vi "Digital Output.vi"(8 "error in":errorcluster, 11 "DAQmx OutPut Setting":T1) -> (0 "error out":errorcluster, 1 "Exit":bool)   [LabVIEW 2015]
uses:
  <vilib>/DAQmx/write.llb/DAQmx Write (Digital 2D Bool NChan 1Samp NLine).vi
  <vilib>/DAQmx/write.llb/DAQmx Write (Digital 1D Bool 1Chan 1Samp).vi
  <vilib>/DAQmx/create/channels.llb/DAQmx Create Channel (DO-Digital Output).vi
  Galobal variable_TI.vi
  <vilib>/DAQmx/miscellaneous.llb/DAQmx Fill In Error Info.vi
panel:
  out "error out 2":errorcluster
  out "array":tag[](array[tag])
  out "*(type *) &x":tag
  out "Digital Output":bool[](array[boolean])
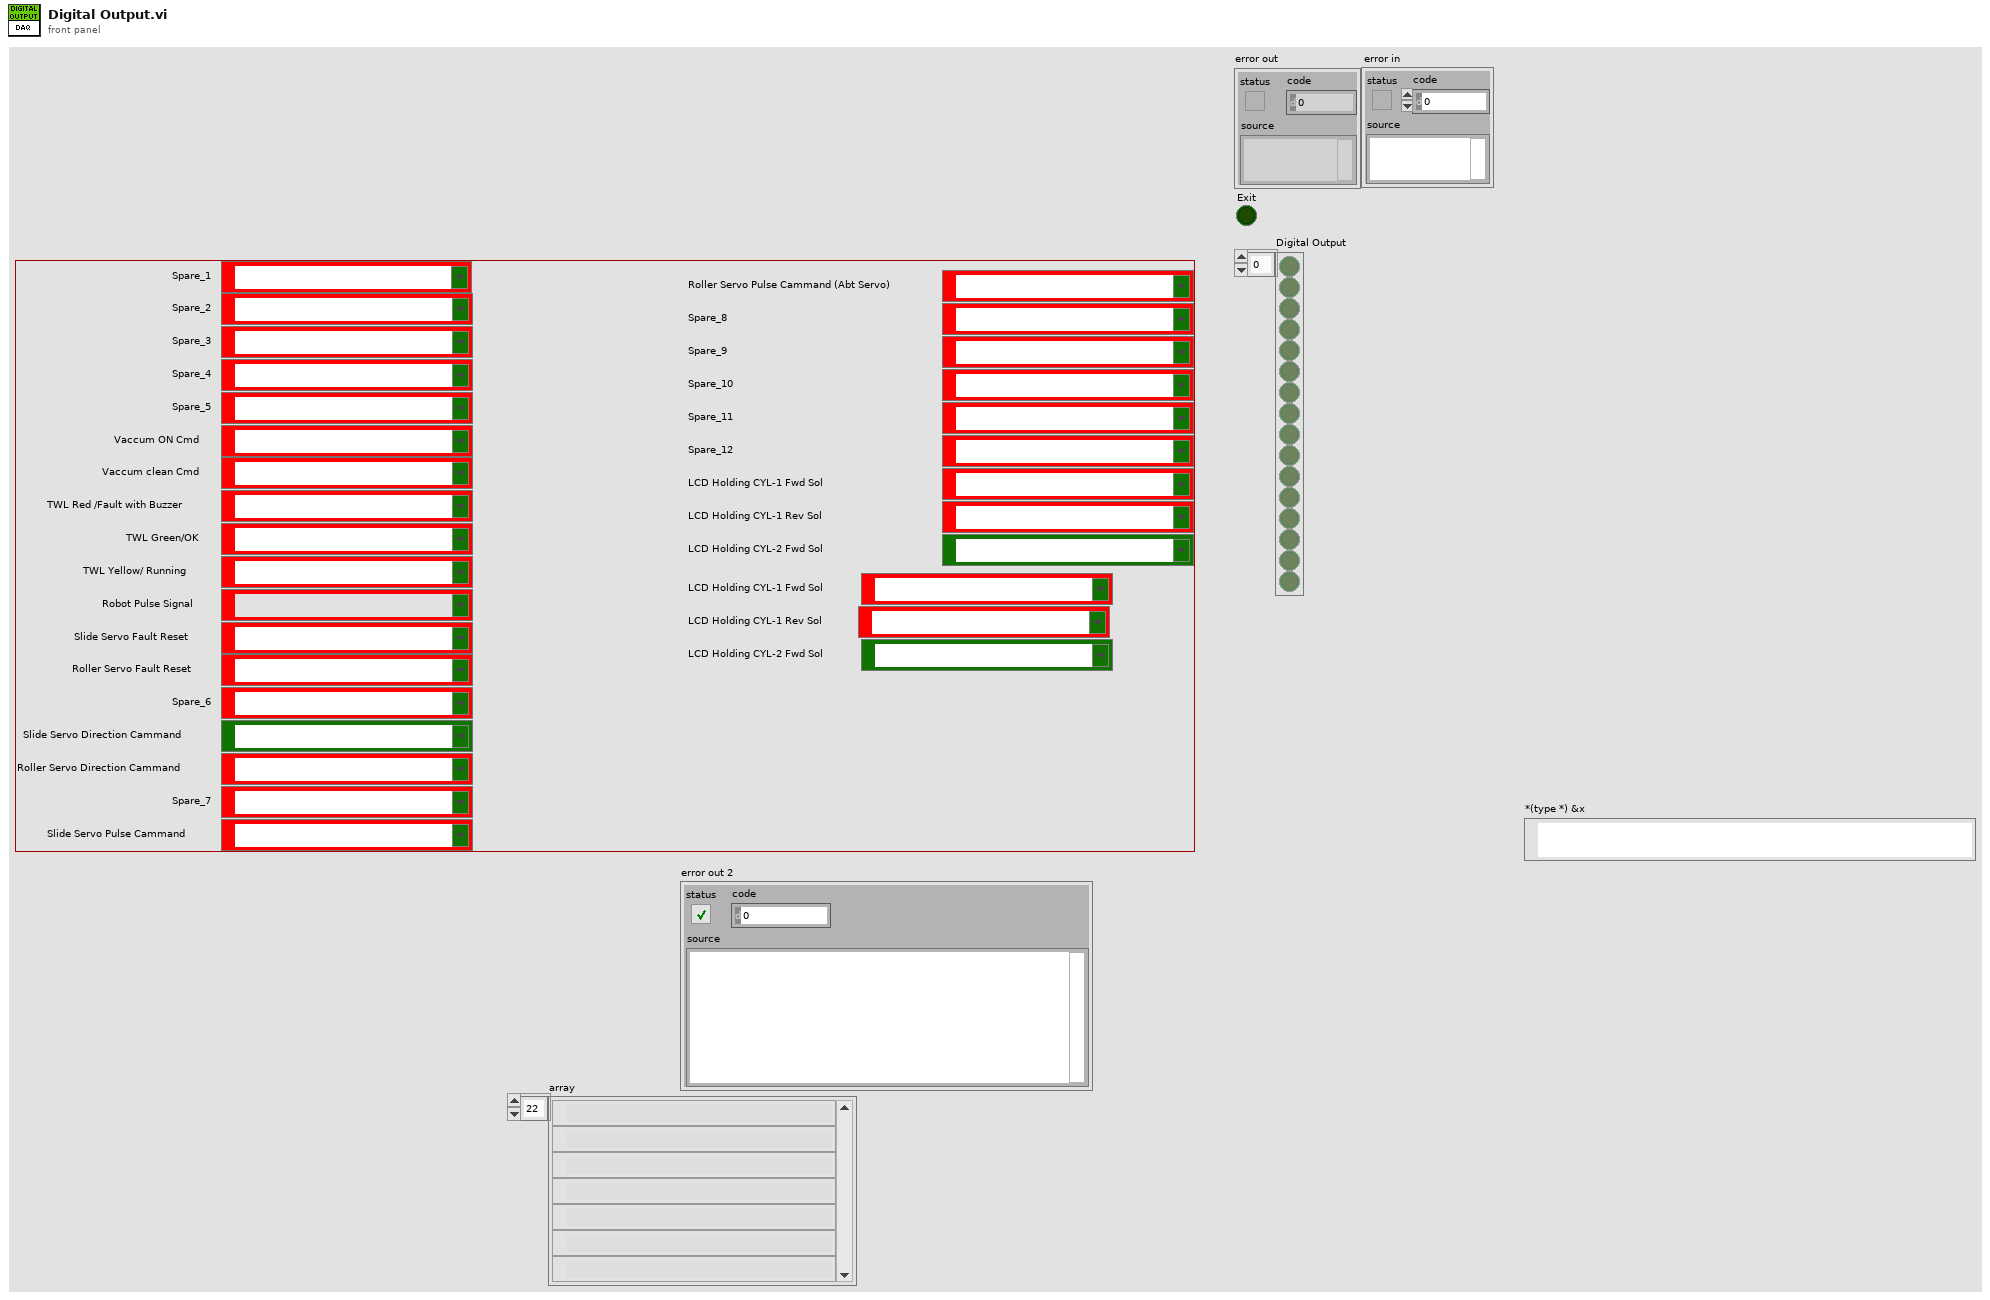
[diagram p1: front panel]
types:
  T1 = cluster{"DAQmx OutPut_00":tag, "DAQmx OutPut_01":tag, "DAQmx OutPut_02":tag, "DAQmx OutPut_03":tag, "DAQmx OutPut_04":tag, "DAQmx OutPut_05":tag, "DAQmx OutPut_06":tag, "DAQmx OutPut_07":tag, "DAQmx OutPut_08":tag, "DAQmx OutPut_09":tag, "DAQmx OutPut_10":tag, "DAQmx OutPut_11":tag, "DAQmx OutPut_12":tag, "DAQmx OutPut_13":tag, "DAQmx OutPut_14":tag, "DAQmx OutPut_15":tag, "DAQmx OutPut_16":tag, "DAQmx OutPut_17":tag, "DAQmx OutPut_18":tag, "DAQmx OutPut_19":tag, "DAQmx OutPut_20":tag, "DAQmx OutPut_21":tag, "DAQmx OutPut_22":tag, "DAQmx OutPut_23":tag, "DAQmx OutPut_12 2":tag, "DAQmx OutPut_13 2":tag, "DAQmx OutPut_14 2":tag, "DAQmx OutPut_12 3":tag, "DAQmx OutPut_13 3":tag, "DAQmx OutPut_14 3":tag}
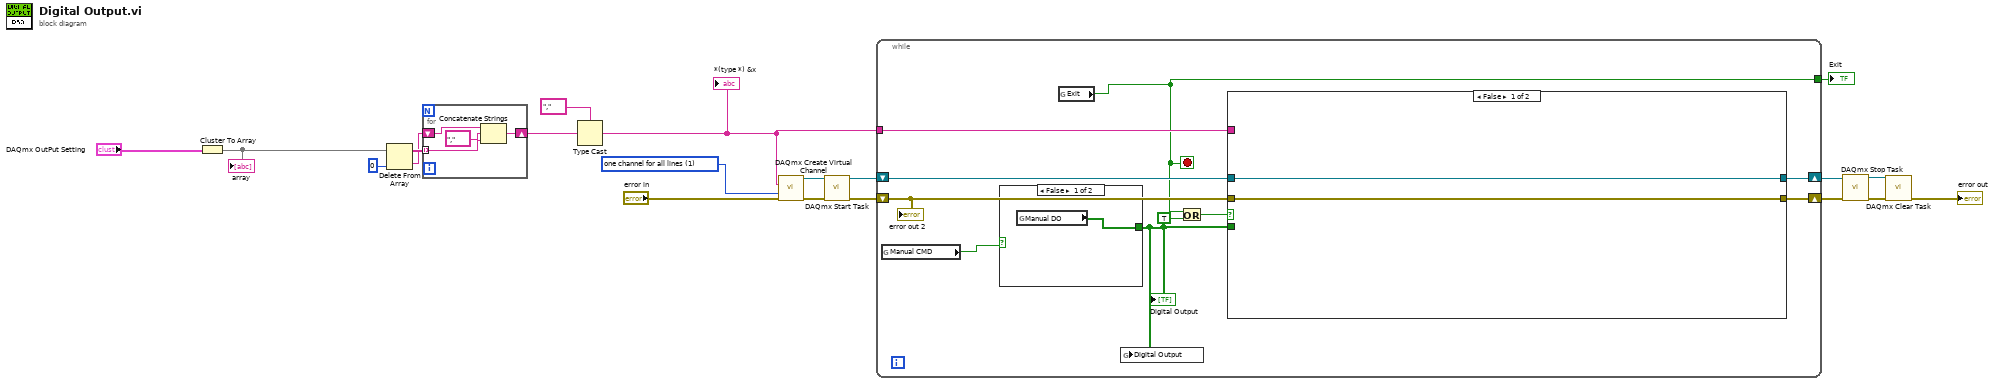
[diagram p0: block diagram]
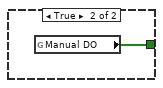
[diagram p2: hidden frame]
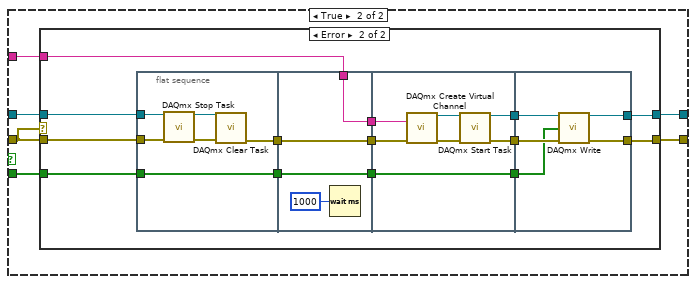
[diagram p3: hidden frame]
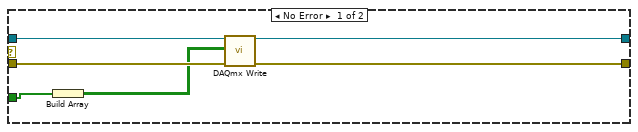
[diagram p4: hidden frame]
diagram:
  w4 = 1 items=["one channel for each line", "one channel for all lines"] ("line grouping")
  n1 = Cluster To Array(cluster="DAQmx OutPut Setting") -> (array=w2:tag[])
  "array" <- w2
  n2 = Delete From Array(array=w2, index=0) -> (deleted portion=w7:tag, array with subset deleted=w9:tag[])  [unwired: 1 in]
  n3 = for {
    tunnel: w9 -> [w23] mode=indexing
    shift-right: [w21] -> w5
    shift-left: w7 -> [w24]
    n4 = Concatenate Strings(w24, tag "," ("1."), w23) -> (w21:string)
  }
  n5 = Type Cast(type=tag "," ("1."), x=w5) -> (*(type *) &x=w3:tag)
  "*(type *) &x" <- w3
  n6 = call-poly <vilib>:"DAQmx Create Virtual Channel.vi"("lines"=w3, "line grouping"=w4, "error in"="error in") -> ("task out"=w20:refnum<k21>, "error out"=w19:errorcluster)  [unwired: 2 in, 9 out]
  n7 = call <vilib>:"DAQmx Start Task.vi"("task/channels in"=w20, "error in"=w19) -> ("task out"=w16:refnum<k21>, "error out"=w15:errorcluster)  [unwired: 12 out]
  n8 = while {
    shift-right: [w32] -> w13
    shift-left: w15 -> [w31]
    shift-right: [w33] -> w14
    shift-left: w16 -> [w34]
    tunnel: w3 -> [w30]
    tunnel: [w27] -> w10
    stop <- w27 stop-if-true
    n9 = global read "Galobal variable_TI.vi" "Manual CMD"() -> (w26:bool)
    n10 = case shown="False" w26 {
      tunnel: [w35 w36] -> w25
      frame False {
        n11 = global read "Galobal variable_TI.vi" "Manual DO"() -> (w35:bool[])
      }
      frame True {
        n12 = global read "Galobal variable_TI.vi" "Manual DO"() -> (w36:bool[])
      }
    }
    "Digital Output" <- w25
    n13 = global read "Galobal variable_TI.vi" "Exit"() -> (w27:bool)
    n14 = global write "Galobal variable_TI.vi" "Digital Output"(w25) -> ()
    n15 = Or(x=w27, y=TRUE) -> (x .or. y?=w29:bool)
    n16 = case shown="False" w29 {
      tunnel: w34 -> [w38 w44]
      tunnel: [w38 w43] -> w33
      tunnel: [w37 w42] -> w32
      tunnel: w31 -> [w37 w41]
      tunnel: w30 -> [_ w40]
      tunnel: w25 -> [_ w39]
      frame False {
      }
      frame True {
        n17 = case shown="Error" w41 {
          tunnel: w44 -> [w50 w64]
          tunnel: w41 -> [w49 w63]
          tunnel: [w48 w61] -> w43
          tunnel: [w47 w62] -> w42
          tunnel: w40 -> [_ w57]
          tunnel: w39 -> [w46 w54]
          frame No Error {
            n18 = Build Array(w46) -> (w45:bool[][])
            n19 = call-poly <vilib>:"DAQmx Write.vi"("task/channels in"=w50, "data"=w45, "error in"=w49) -> ("task out"=w48:refnum<k21>, "error out"=w47:errorcluster)  [unwired: 1 in, 10 out]
          }
          frame Error {
            n20 = flat-sequence {
              tunnel: w64 -> [w68]
              tunnel: w63 -> [w67]
              tunnel: [w66] -> w59
              tunnel: w54 -> [w65]
              tunnel: [w65] -> w53
              tunnel: [w73] -> w60
              tunnel: w59 -> [w73]
              tunnel: [w72] -> w58
              tunnel: w57 -> [w72]
              tunnel: w53 -> [w71]
              tunnel: [w71] -> w52
              tunnel: w60 -> [w77]
              tunnel: w58 -> [w76]
              tunnel: [w79] -> w56
              tunnel: [w78] -> w55
              tunnel: w52 -> [w75]
              tunnel: [w75] -> w51
              tunnel: [w84] -> w61
              tunnel: [w85] -> w62
              tunnel: w56 -> [w86]
              tunnel: w55 -> [w83]
              tunnel: w51 -> [w82]
              frame #0 {
                n21 = call <vilib>:"DAQmx Stop Task.vi"("task/channels in"=w68, "error in"=w67) -> ("task out"=w69:refnum<k21>, "error out"=w70:errorcluster)  [unwired: 12 out]
                n22 = call <vilib>:"DAQmx Clear Task.vi"("task in"=w69, "error in"=w70) -> ("error out"=w66:errorcluster)  [unwired: 13 out]
              }
              frame #1 {
                n23 = Wait (ms)(milliseconds to wait=u32 1000) -> ()  [unwired: 1 out]
              }
              frame #2 {
                n24 = call-poly <vilib>:"DAQmx Create Virtual Channel.vi"("lines"=w76, "error in"=w77) -> ("task out"=w81:refnum<k21>, "error out"=w80:errorcluster)  [unwired: 3 in, 9 out]
                n25 = call <vilib>:"DAQmx Start Task.vi"("task/channels in"=w81, "error in"=w80) -> ("task out"=w78:refnum<k21>, "error out"=w79:errorcluster)  [unwired: 12 out]
              }
              frame #3 {
                n26 = call-poly <vilib>:"DAQmx Write.vi"("task/channels in"=w83, "data"=w82, "error in"=w86) -> ("task out"=w84:refnum<k21>, "error out"=w85:errorcluster)  [unwired: 1 in, 10 out]
              }
            }
          }
        }
      }
    }
    "error out 2" <- w31
  }
  "Exit" <- w10
  n27 = call <vilib>:"DAQmx Stop Task.vi"("task/channels in"=w14, "error in"=w13) -> ("task out"=w18:refnum<k21>, "error out"=w17:errorcluster)  [unwired: 12 out]
  n28 = call <vilib>:"DAQmx Clear Task.vi"("task in"=w18, "error in"=w17) -> ("error out"=→"error out":errorcluster)  [unwired: 13 out]
